vi "Get Columns.vi"(9 "Graph ref":refnum<vi>, 10 "Lines":i32, 11 "Refnum in":T1) -> (1 "Points":cluster{cluster{dbl, dbl}, cluster{dbl, dbl}}[](array[cluster]), 2 "Pixels (U16)":u16[][](array[numeric]), 3 "Refnum in 2":T1)   [LabVIEW 2017]
uses:
  <vilib>/vision/Image Controls.llb/IMAQ Image.ctl
  <vilib>/vision/NI_Vision_Development_Module.lvlib
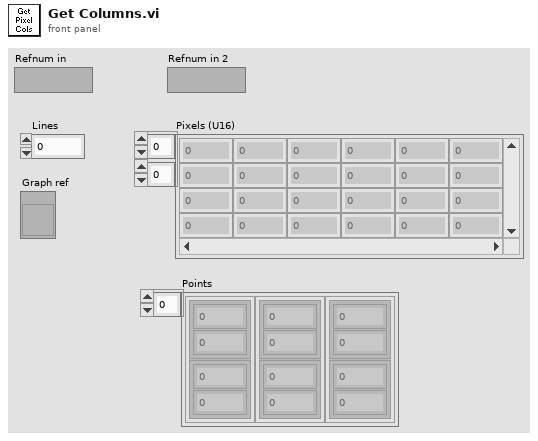
[diagram p1: front panel]
types:
  T1 = typedef "IMAQ Image.ctl" = refnum<image>
  T2 = cluster{cluster{"y":dbl, "y":dbl}, cluster{i32, "y":dbl}}
  T3 = cluster{cluster{"y":dbl, i32}, cluster{i32, i32}}
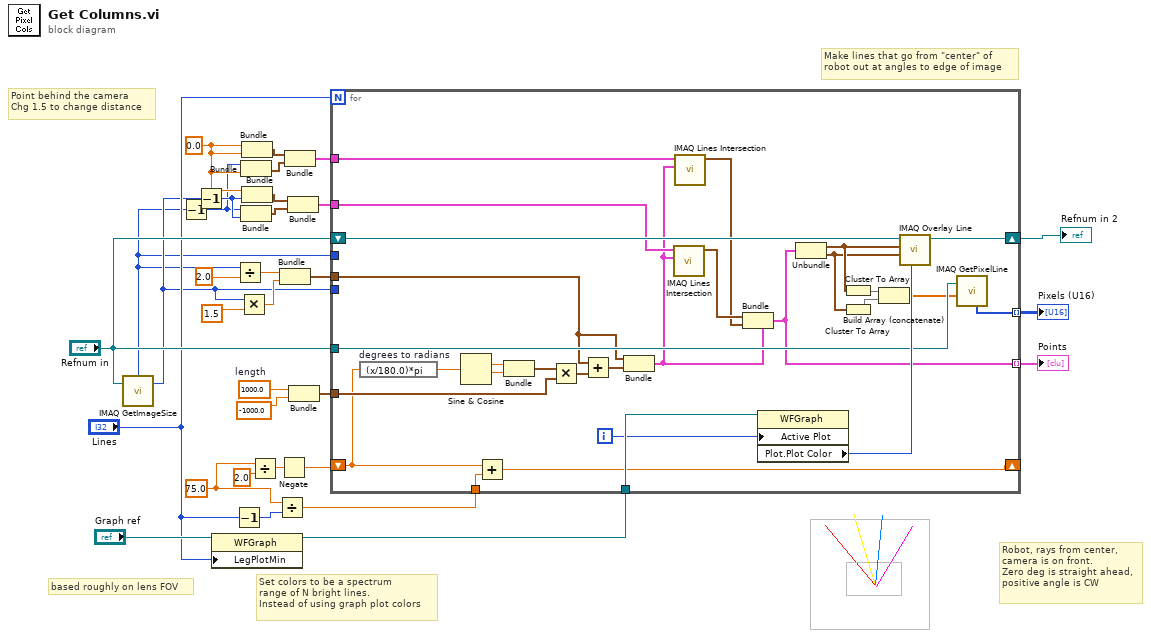
[diagram p0: block diagram]
diagram:
  w8 = 0.0 ("y")
  w18 = 1000.0  # length
  w26 = 75.0 ("y")
  # "Robot, rays from center,\ncamera is on front.\nZero deg is straight ahead,\npositive angle is CW"
  # "Point behind the camera\nChg 1.5 to change distance"
  # "based roughly on lens FOV"
  # "Set colors to be a spectrum\nrange of N bright lines.\nInstead of using graph plot colors"
  # "Make lines that go from \"center\" of\nrobot out at angles to edge of image"
  n1 = call "IMAQ GetImageSize"("Image"="Refnum in") -> ("Y Resolution"=w4:i32, "X Resolution"=w3:i32)  [unwired: 3 in, 1 out]
  n2 = Decrement(x=w3) -> (x-1=w1:i32)
  n3 = Decrement(x=w4) -> (x-1=w2:i32)
  n4 = property class="WFGraph"(reference="Graph ref", "LegPlotMin"="Lines") -> (reference out=w13:refnum<vi>)  [unwired: 1 in, 1 out]
  n5 = Decrement(x="Lines") -> (x-1=w29:i32)
  n6 = Divide(x=w3, y=2.0) -> (x/y=w21:dbl)
  n7 = Multiply(x=w4, y=1.5) -> (x*y=w20:dbl)
  n8 = Bundle(w1, "y"=w8) -> (w6:cluster{i32, "y":dbl})  [unwired: 1 in]
  n9 = Bundle(w1, w2) -> (w10:cluster{i32, i32})  [unwired: 1 in]
  n10 = Bundle("y"=w8, "y"=w8) -> (w7:cluster{"y":dbl, "y":dbl})  [unwired: 1 in]
  n11 = Bundle("y"=w8, w2) -> (w11:cluster{"y":dbl, i32})  [unwired: 1 in]
  n12 = Divide(x=w26, y=2.0) -> (x/y=w24:dbl)
  n13 = Divide(x=w26, y=w29) -> (x/y=w28:dbl)
  n14 = Negate(x=w24) -> (-x=w25:dbl)
  n15 = Bundle(w21, w20) -> (w19:cluster{dbl, dbl})  [unwired: 1 in]
  n16 = Bundle(w7, w6) -> (w5:T2)  [unwired: 1 in]
  n17 = Bundle(w11, w10) -> (w9:T3)  [unwired: 1 in]
  n18 = Bundle("length"=w18, "y"=-1000.0) -> (w16:cluster{"length":dbl, "y":dbl})  [unwired: 1 in]
  n19 = for {
    N: "Lines" -> [_]
    tunnel: "Refnum in" -> [w56]
    tunnel: [w47] -> w30 mode=indexing
    shift-right: [w60] -> w31
    shift-left: "Refnum in" -> [w61]
    tunnel: w4 -> [_]
    tunnel: w13 -> [w59]
    shift-right: [w54] -> _
    shift-left: w25 -> [w45]
    tunnel: w28 -> [w55]
    tunnel: w19 -> [w46]
    tunnel: w16 -> [w51]
    tunnel: [w36] -> w15 mode=indexing
    tunnel: w3 -> [_]
    tunnel: w9 -> [w38]
    tunnel: w5 -> [w35]
    i -> [w58]
    n20 = expression code="(x/180.0)*pi" "degrees to radians"(w45) -> (w44:dbl)
    n21 = Sine & Cosine(0:w44) -> (1:w49:dbl, 2:w50:dbl)
    n22 = Add(x=w45, y=w55) -> (x+y=w54:dbl)
    n23 = Bundle(w49, w50) -> (w53:cluster{dbl, dbl})  [unwired: 1 in]
    n24 = Multiply(x=w53, y=w51) -> (x*y=w52:cluster{dbl, dbl})
    n25 = Add(x=w46, y=w52) -> (x+y=w48:cluster{dbl, dbl})
    n26 = Bundle(w46, w48) -> (w34:cluster{cluster{dbl, dbl}, cluster{dbl, dbl}})  [unwired: 1 in]
    n27 = call "IMAQ Lines Intersection"("Line 2"=w34, "Line 1"=w38) -> ("Intersection Point"=w37:cluster{"X":sgl, "Y":sgl})  [unwired: 7 in, 2 out]
    n28 = call "IMAQ Lines Intersection"("Line 2"=w34, "Line 1"=w35) -> ("Intersection Point"=w33:cluster{"X":sgl, "Y":sgl})  [unwired: 7 in, 2 out]
    n29 = Bundle(cluster=w34, w37, w33) -> (w36:cluster{cluster{dbl, dbl}, cluster{dbl, dbl}})
    n30 = property class="WFGraph"(reference=w59, "Active Plot"=w58) -> ("Plot.Plot Color"=w57:u32)  [unwired: 1 in, 2 out]
    n31 = Unbundle(w36) -> (w43:cluster{dbl, dbl}, w42:cluster{dbl, dbl})
    n32 = Cluster To Array(cluster=w43) -> (array=w41:dbl[])
    n33 = Cluster To Array(cluster=w42) -> (array=w40:dbl[])
    n34 = Build Array (concatenate)(w41, w40) -> (w39:dbl[])
    n35 = call "IMAQ Overlay Line"("Color"=w57, "End Point"=w42, "Start Point"=w43, "Image"=w61) -> ("Image Out"=w60:T1)  [unwired: 6 in, 1 out]
    n36 = call "IMAQ GetPixelLine"("Line Coordinates"=w39, "Image"=w56) -> ("Pixels Line (U16)"=w47:u16[])  [unwired: 2 in, 4 out]
  }
  "Pixels (U16)" <- w30
  "Refnum in 2" <- w31
  "Points" <- w15
